vi "getData.vi"(8 "error in (no error)":errorcluster, 11 "rf in":refnum<class "rf.lvclass">) -> (0 "error out":errorcluster, 1 "dataType":T1(ring), 2 "data":T2, 3 "rf out":refnum<class "rf.lvclass">)   [LabVIEW 2009, in "Tools.lvlib" / "Scripting.lvlib" / "rf.lvclass"]
uses:
  rf.lvclass
  DatabaseHelpers/Database Objects/Channel/Channel.lvclass
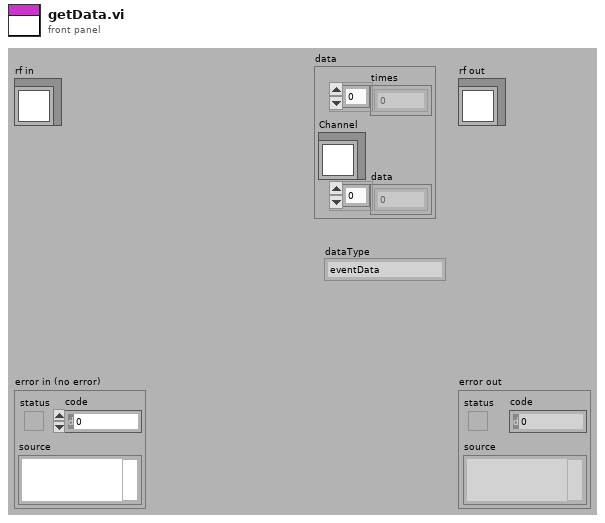
[diagram p1: front panel]
types:
  T1 = enum16{"eventData", "singleToneData", "fileData"}
  T2 = cluster{"times":dbl[], "Channel":refnum<class "Channel.lvclass">, "data":dbl[]}
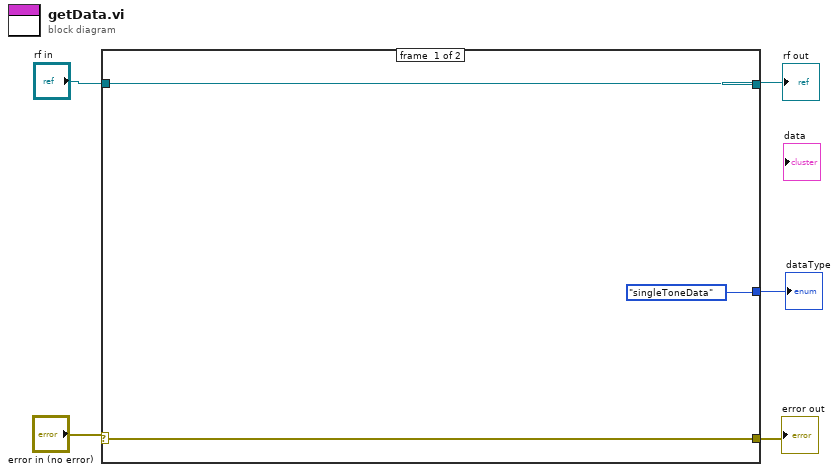
[diagram p0: block diagram]
diagram:
  n1 = case shown="No Error" "error in (no error)" {
    selector: "error in (no error)" -> [w7 w9]
    tunnel: [w8 w10] -> w5
    tunnel: "rf in" -> [w8 w10]
    tunnel: [w7 w9] -> w2
    tunnel: [T1."singleToneData" ("dataType") _] -> w1
    frame #0 {
    }
    frame #1 {
    }
  }
  "error out" <- w2
  "rf out" <- w5
  "dataType" <- w1
